vi "Draw Rangefinder.vi"(5 "FcdVI Refnum":refnum<vi>, 7 "2D Picture":refnum<vi>, 9 "State":T1={"Draw Options"={"Background Color"=16777215, "Grid Color"=13816530, "Angle Units"=enum."Radians", "Draw Solid Background"=TRUE, "Draw Grid"=TRUE, "Grid Spacing"=1.0, "AutoScale"=TRUE, "Fit to Radius"=1.0, "data row options"=[]}}, 10 "data":T5) -> (3 "Picture Out":picture)   [LabVIEW 2017, in "NI_Robotics_2D Rangefinder.xctl"]
uses:
  <vilib>/robotics/Controls/2D Rangefinder/NI_Robotics_2D Rangefinder.xctl
  <vilib>/robotics/Controls/2D Rangefinder/_2D Rangefinder Support Files/Data.ctl
  <vilib>/robotics/Controls/2D Rangefinder/_2D Rangefinder Support Files/State.ctl
  <vilib>/robotics/Controls/2D Rangefinder/2D Rangefinder Picture/Draw Options.ctl
  <vilib>/robotics/Controls/Utilities/Angle Units.ctl
  <vilib>/robotics/Controls/2D Rangefinder/2D Rangefinder Picture/Data Row Options.ctl
  <vilib>/Utility/miscctls.llb/LVBoundsTypeDef.ctl
  <vilib>/Utility/miscctls.llb/LVPositionTypeDef.ctl
  <vilib>/robotics/Controls/2D Rangefinder/2D Rangefinder Picture/NI_Robotics_2D Rangefinder Picture.lvlib
  <vilib>/robotics/Controls/Utilities/NI_Robotics_Control Utilities.lvlib
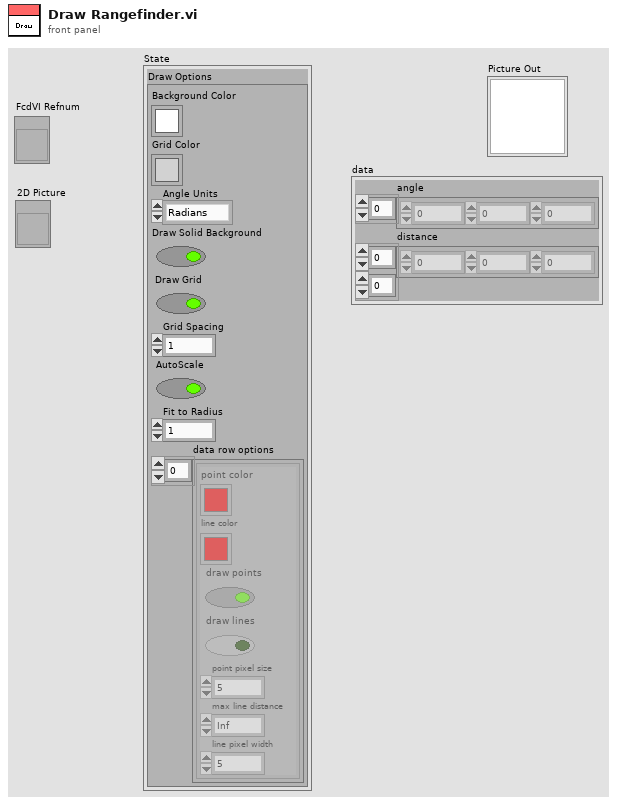
[diagram p1: front panel]
types:
  T1 = typedef "NI_Robotics_2D Rangefinder.xctl/State.ctl" = cluster{"Draw Options":T2}
  T2 = typedef "NI_Robotics_2D Rangefinder Picture.lvlib/Draw Options.ctl" = cluster{"Background Color":u32, "Grid Color":u32, "Angle Units":T3, "Draw Solid Background":bool, "Draw Grid":bool, "Grid Spacing":dbl, "AutoScale":bool, "Fit to Radius":dbl, "data row options":T4[]}
  T3 = typedef "NI_Robotics_Control Utilities.lvlib/Angle Units.ctl" = enum16{"Radians", "Degrees"}
  T4 = typedef "NI_Robotics_2D Rangefinder Picture.lvlib/Data Row Options.ctl" = cluster{"point color":u32, "line color":u32, "draw points":bool, "draw lines":bool, "point pixel size":u16, "max line distance":dbl, "line pixel width":u16}
  T5 = typedef "NI_Robotics_2D Rangefinder.xctl/Data.ctl" = cluster{"angle":dbl[], "distance":dbl[][]}
  T6 = typedef "LVPositionTypeDef.ctl" = cluster{"Left":i32, "Top":i32}
  T7 = typedef "LVBoundsTypeDef.ctl" = cluster{"Width":u32, "Height":u32}
  T8 = typedef "LVRectTypeDef.ctl" = cluster{"Left":i16, "Top":i16, "Right":i16, "Bottom":i16}
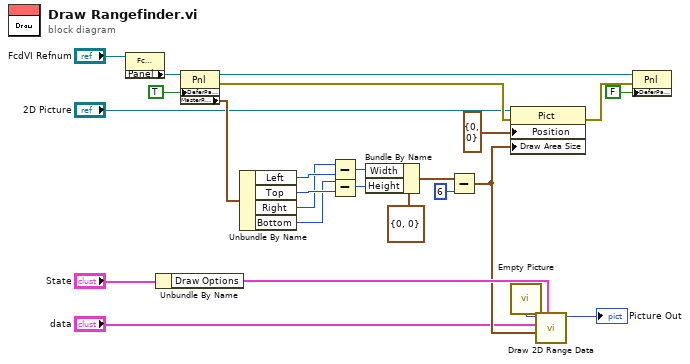
[diagram p0: block diagram]
diagram:
  n1 = property class="FcdVI"(reference="FcdVI Refnum") -> ("Panel"=w5:refnum<vi>)  [unwired: 1 in, 2 out]
  n2 = Unbundle By Name("State") -> ("Draw Options"=w23:T2)
  n3 = property class="Pnl"(reference=w5, "DeferPanUpdts"=TRUE ("Defer Panel Updates")) -> (reference out=w7:refnum<vi>, error out=w9:errorcluster, "MasterRect"=w11:T8)  [unwired: 1 in]
  n4 = Unbundle By Name(w11) -> ("Left"=w13:i16, "Top"=w15:i16, "Right"=w12:i16, "Bottom"=w14:i16)
  n5 = Subtract(x=w12, y=w13) -> (x-y=w17:i16)
  n6 = Subtract(x=w14, y=w15) -> (x-y=w18:i16)
  n7 = Bundle By Name(cluster=T7 {"Width"=0, "Height"=0} ("Draw Area Size"), "Width"=w17, "Height"=w18) -> (w19:T7)
  n8 = Subtract(x=w19, y=u32 6) -> (x-y=w2:T7)
  n9 = property class="Pict"(reference="2D Picture", error in=w9, "Position"=T6 {"Left"=0, "Top"=0}, "Draw Area Size"=w2) -> (error out=w10:errorcluster)  [unwired: 1 out]
  n10 = call "Empty Picture"() -> ("empty picture"=w25:picture)
  n11 = call <vilib>:"Draw 2D Range Data.vi"("draw options"=w23, "DrawAreaSize"=w2, "data"="data", "picture in"=w25) -> ("picture out"=→"Picture Out":picture)  [unwired: 6 in, 1 out]
  n12 = property class="Pnl"(reference=w7, error in=w10, "DeferPanUpdts"=FALSE ("Defer Panel Updates")) -> ()  [unwired: 2 out]
